vi "channeldata_timestamp_interleaved.vi"() -> ()   [LabVIEW 2019]
panel:
  out "Error Out":errorcluster
  in  "TDMS File":path=path "C:/Python/projects/nitdms/tests/tdms_files/channeldata_timestamp_interleaved.tdms"
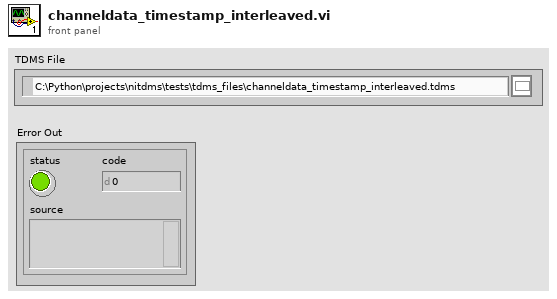
[diagram p1: front panel]
types:
  T1 = enum16{"open", "open or create", "create or replace", "create", "open (read-only)"}
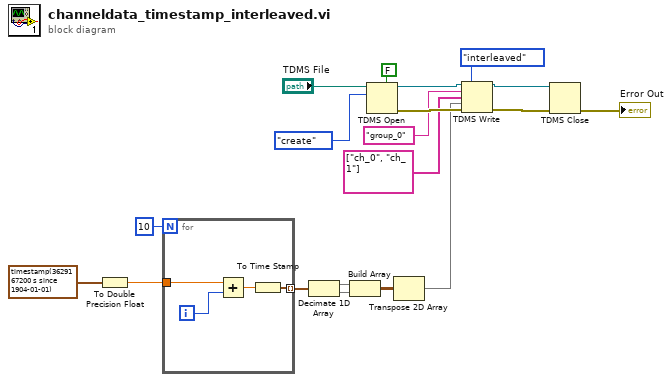
[diagram p0: block diagram]
diagram:
  n1 = To Double Precision Float(number=timestamp(3629167200 s since 1904-01-01)) -> (double precision float=w8:dbl)
  n2 = for {
    N: 10 -> [_]
    tunnel: w8 -> [w23]
    tunnel: [w20] -> w5 mode=indexing
    i -> [w22]
    n3 = Add(x=w23, y=w22) -> (x+y=w21:dbl)
    n4 = To Time Stamp(1:w21) -> (0:w20:timestamp)
  }
  n5 = Decimate 1D Array(w5) -> (w4:timestamp[], w3:timestamp[])
  n6 = Build Array(w4, w3) -> (w2:timestamp[][])
  n7 = TDMS Open(5:FALSE ("create index file? (T)"), 10:T1."create" ("operation (0:open)"), 11:"TDMS File") -> (0:w15:errorcluster, 3:w14:refnum<k34>)  [unwired: 4 in]
  n8 = Transpose 2D Array(2D array=w2) -> (transposed array=w1:timestamp[][])
  n9 = TDMS Write(0:w14, 1:enum16{"decimated", "interleaved"}."interleaved" ("data layout (0:decimated)"), 5:"group_0", 7:string[] ["ch_0", "ch_1"], 9:w1, 11:w15) -> (4:w12:refnum<k34>, 15:w13:errorcluster)  [unwired: 2 out]
  n10 = TDMS Close(8:w13, 11:w12) -> (0:→"Error Out":errorcluster)  [unwired: 1 out]
